vi "PH_PSDBWriter.set GUI Refs.vi"(0 "i ref in":refnum<vi>, 1 "Class":string, 2 "Ref PSDB Status":refnum<vi>, 5 "error in":errorcluster) -> (14 "i ref out":refnum<vi>, 19 "error out":errorcluster)   [LabVIEW 2014, in "PH_PSDBWriter.lvlib"]
doc: "This VI sets the relevant GUI references to own attributes."
uses:
  PH_PSDBWriter.lvlib
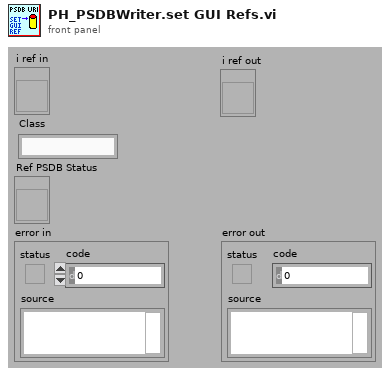
[diagram p1: front panel]
types:
  T1 = typedef "PH_PSDBWriter.lvlib/PH_PSDBWriter.i attribute.ctl" = cluster{"PSDB Status Service ID":i32, "Instance ID":i32, "Shot #":i32, "Subsystem":T2, "Data Status":T3, "Ref PSDB Status":refnum<vi>, "PSDB Error Code":i32, "PSDB Dataset":T4, "PSDB Thread":cluster{"Ref":refnum<vi>, "Q-Ref":refnum<queue>}, "PSDB Credentials":T12}
  T2 = typedef "PH_PSDBWriter.lvlib/PH_PSDBWriter.PHELIX-Subsystems.ctl" = i32
  T3 = typedef "PH_PSDBWriter.lvlib/PH_PSDBWriter.Data Status.ctl" = i16
  T4 = typedef "PH_PSDBWriter.lvlib/PH_PSDBWriter.PSDB Dataset.ctl" = cluster{"Version":i32, "2D data Input":T5[], "Boolean Input":T7[], "Image Input":T8[], "Numeric Input":T10[], "String Input":T11[]}
  T5 = typedef "PH_PSDBWriter.lvlib/PH_PSDBWriter.2D dataset.ctl" = cluster{"name":string, "data":dbl[][], "axis description":T6}
  T6 = typedef "PSDB.lvlib/PSDB_AxisDescription.ctl" = cluster{"x axis label":string, "y axis label":string, "x axis unit":string, "y axis unit":string}
  T7 = typedef "PH_PSDBWriter.lvlib/PH_PSDBWriter.Boolean dataset.ctl" = cluster{"name":string, "data":bool, "unit":string}
  T8 = typedef "PH_PSDBWriter.lvlib/PH_PSDBWriter.Image dataset.ctl" = cluster{"name":string, "data":T9, "unit":string}
  T9 = typedef "IMAQ Image.ctl" = refnum<image>
  T10 = typedef "PH_PSDBWriter.lvlib/PH_PSDBWriter.Numeric dataset.ctl" = cluster{"name":string, "data":dbl, "unit":string}
  T11 = typedef "PH_PSDBWriter.lvlib/PH_PSDBWriter.String dataset.ctl" = cluster{"name":string, "data":string, "unit":string}
  T12 = typedef "PH_Common.lvlib/PH_Connection.PSDB Credentials.ctl" = cluster{"PW":string, "ID":string, "DS":string}
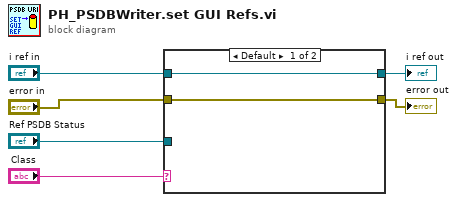
[diagram p0: block diagram]
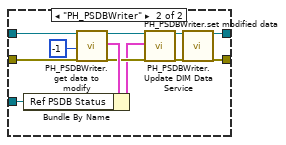
[diagram p2: hidden frame]
diagram:
  n1 = case shown="Default" "Class" {
    tunnel: "Ref PSDB Status" -> [_ w19]
    tunnel: "error in" -> [w7 w17]
    tunnel: "i ref in" -> [w8 w15]
    tunnel: [w7 w9] -> w3
    tunnel: [w8 w10] -> w2
    frame Default {
    }
    frame "PH_PSDBWriter" {
      n2 = call "PH_PSDBWriter.get data to modify.vi"("i ref in"=w15, "ms timeout (10000)"=-1, "error in (no error)"=w17) -> ("i ref out"=w14:refnum<vi>, "i attribute"=w18:T1, "error out"=w16:errorcluster)  [unwired: 13 in, 1 out]
      n3 = Bundle By Name(cluster=w18, "Ref PSDB Status"=w19) -> (w11:T1)
      n4 = call "PH_PSDBWriter.set modified data.vi"("i ref in"=w14, "i attribute"=w11, "error in (no error)"=w16) -> ("i ref out"=w13:refnum<vi>, "error out"=w12:errorcluster)  [unwired: 15 in]
      n5 = call "PH_PSDBWriter.Update DIM Data Service.vi"("i ref in"=w13, "error in"=w12) -> ("i ref out"=w10:refnum<vi>, "error out"=w9:errorcluster)  [unwired: 16 in]
    }
  }
  "error out" <- w3
  "i ref out" <- w2
